vi "Cargo Manip Control.vi"   [LabVIEW 2018]
uses:
  SubSystems/Cargo Intake/Cargo Intake Global.vi
  SubSystems/Controllers/Manipulator Controlller/Manipulator Controller Global.vi
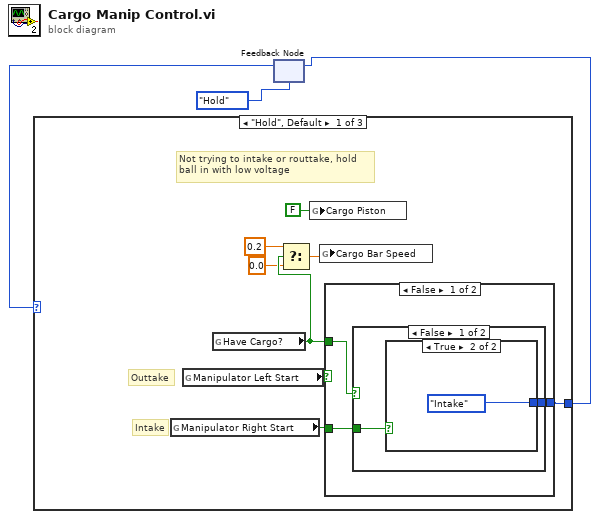
[diagram p0: block diagram]
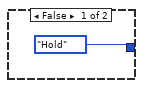
[diagram p2: hidden frame]
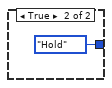
[diagram p3: hidden frame]
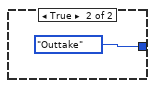
[diagram p4: hidden frame]
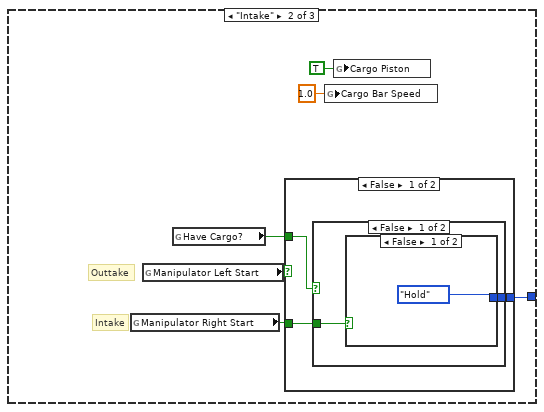
[diagram p5: hidden frame]
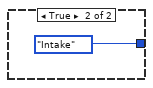
[diagram p6: hidden frame]
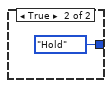
[diagram p7: hidden frame]
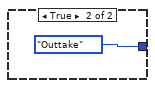
[diagram p8: hidden frame]
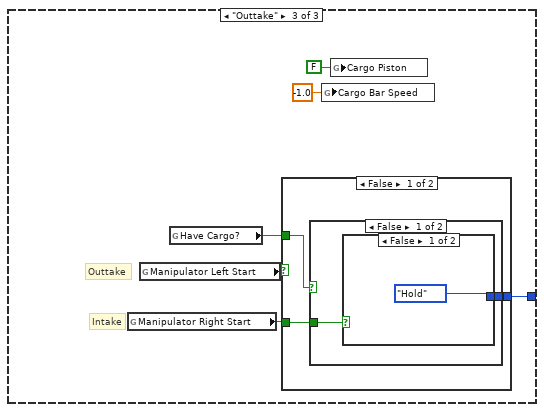
[diagram p9: hidden frame]
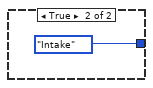
[diagram p10: hidden frame]
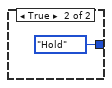
[diagram p11: hidden frame]
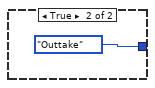
[diagram p12: hidden frame]
diagram:
  n1 = feedback #1(enum16{"Going Up", "Outtake", "Intake", "Hold"}."Hold") -> (w2:enum16{"Going Up", "Outtake", "Intake", "Hold"})
  n2 = case shown="\"Hold\", Default" w2 {
    tunnel: [w9 w21 w36] -> w1
    frame "Hold", Default {
      # "Outtake"
      # "Intake"
      # "Not trying to intake or routtake, hold\nball in with low voltage"
      n3 = global read "Manipulator Controller Global.vi" "Manipulator Right Start"() -> (w11:bool)
      n4 = global read "Manipulator Controller Global.vi" "Manipulator Left Start"() -> (w10:bool)
      n5 = global read "Cargo Intake Global.vi" "Have Cargo?"() -> (w6:bool)
      n6 = Select(t=0.2, s=w6, f=0.0) -> (s? t:f=w7:dbl)
      n7 = global write "Cargo Intake Global.vi" "Cargo Piston"(FALSE ("Cargo Piston")) -> ()
      n8 = global write "Cargo Intake Global.vi" "Cargo Bar Speed"(w7) -> ()
      n9 = case shown="False" w10 {
        tunnel: w11 -> [w14 _]
        tunnel: [w13 enum16{"Going Up", "Outtake", "Intake", "Hold"}."Outtake"] -> w9
        tunnel: w6 -> [w12 _]
        frame False {
          n10 = case shown="False" w12 {
            tunnel: w14 -> [w16 _]
            tunnel: [w15 enum16{"Going Up", "Outtake", "Intake", "Hold"}."Hold"] -> w13
            frame False {
              n11 = case shown="True" w16 {
                tunnel: [enum16{"Going Up", "Outtake", "Intake", "Hold"}."Hold" enum16{"Going Up", "Outtake", "Intake", "Hold"}."Intake"] -> w15
                frame False {
                }
                frame True {
                }
              }
            }
            frame True {
            }
          }
        }
        frame True {
        }
      }
    }
    frame "Intake" {
      # "Outtake"
      # "Intake"
      n12 = global read "Manipulator Controller Global.vi" "Manipulator Right Start"() -> (w26:bool)
      n13 = global read "Manipulator Controller Global.vi" "Manipulator Left Start"() -> (w25:bool)
      n14 = global read "Cargo Intake Global.vi" "Have Cargo?"() -> (w24:bool)
      n15 = case shown="False" w25 {
        tunnel: w26 -> [w29 _]
        tunnel: [w28 enum16{"Going Up", "Outtake", "Intake", "Hold"}."Outtake"] -> w21
        tunnel: w24 -> [w27 _]
        frame False {
          n16 = case shown="False" w27 {
            tunnel: w29 -> [w31 _]
            tunnel: [w30 enum16{"Going Up", "Outtake", "Intake", "Hold"}."Hold"] -> w28
            frame False {
              n17 = case shown="False" w31 {
                tunnel: [enum16{"Going Up", "Outtake", "Intake", "Hold"}."Hold" enum16{"Going Up", "Outtake", "Intake", "Hold"}."Intake"] -> w30
                frame False {
                }
                frame True {
                }
              }
            }
            frame True {
            }
          }
        }
        frame True {
        }
      }
      n18 = global write "Cargo Intake Global.vi" "Cargo Bar Speed"(1.0 ("Cargo Bar Speed")) -> ()
      n19 = global write "Cargo Intake Global.vi" "Cargo Piston"(TRUE ("Cargo Piston")) -> ()
    }
    frame "Outtake" {
      # "Outtake"
      # "Intake"
      n20 = global read "Manipulator Controller Global.vi" "Manipulator Right Start"() -> (w41:bool)
      n21 = global read "Manipulator Controller Global.vi" "Manipulator Left Start"() -> (w40:bool)
      n22 = global read "Cargo Intake Global.vi" "Have Cargo?"() -> (w39:bool)
      n23 = case shown="False" w40 {
        tunnel: w41 -> [w44 _]
        tunnel: [w43 enum16{"Going Up", "Outtake", "Intake", "Hold"}."Outtake"] -> w36
        tunnel: w39 -> [w42 _]
        frame False {
          n24 = case shown="False" w42 {
            tunnel: w44 -> [w46 _]
            tunnel: [w45 enum16{"Going Up", "Outtake", "Intake", "Hold"}."Hold"] -> w43
            frame False {
              n25 = case shown="False" w46 {
                tunnel: [enum16{"Going Up", "Outtake", "Intake", "Hold"}."Hold" enum16{"Going Up", "Outtake", "Intake", "Hold"}."Intake"] -> w45
                frame False {
                }
                frame True {
                }
              }
            }
            frame True {
            }
          }
        }
        frame True {
        }
      }
      n26 = global write "Cargo Intake Global.vi" "Cargo Bar Speed"(-1.0 ("Cargo Bar Speed")) -> ()
      n27 = global write "Cargo Intake Global.vi" "Cargo Piston"(FALSE ("Cargo Piston")) -> ()
    }
  }
  n28 = feedback-in #1(w1) -> ()
